vi "fit_poly.vi"(10 "X in":dbl[](array[numeric]), 11 "Y in":dbl[](array[numeric])) -> (1 "Y":dbl[](array[numeric]), 2 "X":dbl[](array[numeric]), 3 "peak X":dbl)   [LabVIEW 2015]
uses:
  <vilib>/Analysis/6fits.llb/Curve Fitting Criteria.ctl
  <vilib>/Analysis/6fits.llb/General Linear Fit Algorithm.ctl
  <vilib>/Analysis/NI_AALPro.lvlib
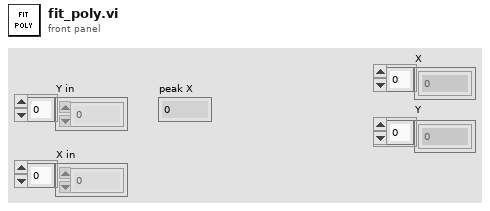
[diagram p1: front panel]
types:
  T1 = typedef "NI_AALPro.lvlib/General Linear Fit Algorithm.ctl" = u16
  T2 = typedef "NI_AALPro.lvlib/Curve Fitting Criteria.ctl" = u16
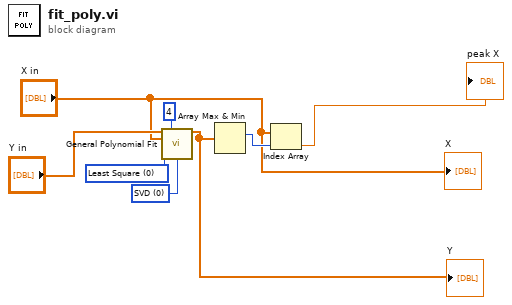
[diagram p0: block diagram]
diagram:
  w3 = T1 0 items=["SVD", "Givens", "Givens2", "Householder", "LU Decomposition", "Cholesky", "SVD for Rank Deficient H"] ("algorithm")
  w2 = T2 0 items=["Least Square", "Least Absolute Residual", "Bisquare"] ("method")
  n1 = call <vilib>:"General Polynomial Fit.vi"("Y"="Y in", "polynomial order"=4, "X"="X in", "method"=w2, "algorithm"=w3) -> ("Best Polynomial Fit"=w7:dbl[])  [unwired: 7 in, 3 out]
  "Y" <- w7
  n2 = Array Max & Min(array=w7) -> (max index (indices)=w5:i32)  [unwired: 3 out]
  n3 = Index Array(array="X in", index=w5) -> (element=→"peak X":dbl)
  "X" <- "X in"
